vi "GetSensorList.vi"(8 "Error In":errorcluster, 11 "Station Id":string) -> (0 "Error Out":errorcluster, 2 "Sensor List":string[](array[string]), 3 "Sensor Id":dbl[](array[numeric]))   [LabVIEW 2020]
doc: "This VI use GET method to get list of sensors and measuring parameters"
uses:
  <vilib>/httpClient/LabVIEWHTTPClient.lvlib
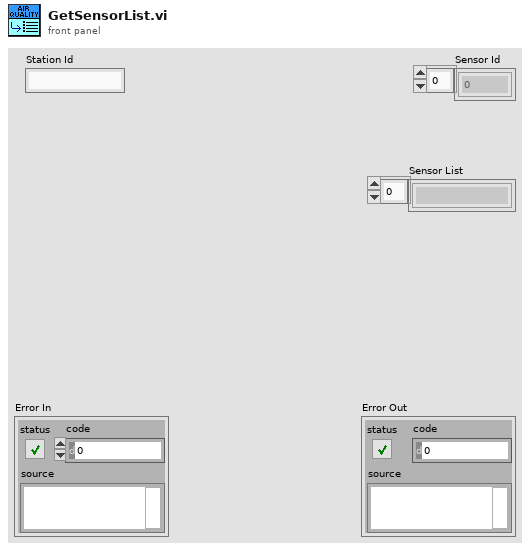
[diagram p1: front panel]
types:
  T1 = cluster{"id":dbl, "stationId":dbl, "param":cluster{"paramName":string, "paramFormula":string, "paramCode":string, "idParam":dbl}}[]
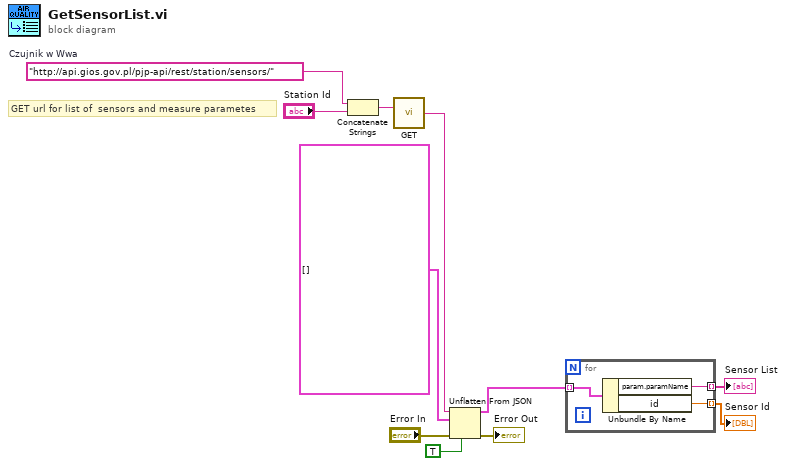
[diagram p0: block diagram]
diagram:
  w9 = "http://api.gios.gov.pl/pjp-api/rest/station/sensors/"  # Czujnik w Wwa
  # "GET url for list of  sensors and measure parametes"
  n1 = Concatenate Strings(w9, "Station Id") -> (w8:string)
  n2 = call <vilib>:"GET.vi"("url"=w8) -> ("body"=w11:string)  [unwired: 11 in, 3 out]
  n3 = Unflatten From JSON(JSON string=w11, type and defaults=T1 [], default null elements? (F)=TRUE, error in (no error)="Error In") -> (value=w4:T1, error out=→"Error Out":errorcluster)  [unwired: 3 in]
  n4 = for {
    tunnel: w4 -> [w14] mode=indexing
    tunnel: [w13] -> w3 mode=indexing
    tunnel: [w12] -> w2 mode=indexing
    n5 = Unbundle By Name(w14) -> ("param.paramName"=w13:string, "id"=w12:dbl)
  }
  "Sensor List" <- w3
  "Sensor Id" <- w2
